vi "Top_Level_Control_Cavities_Pulses_v00.vi"() -> ()   [LabVIEW 2010]
doc: "Provides user interface for `Cavities_Pulse_FPGA_v00.vi'."
uses:
  Strict Type Defs/Control GUI v01.ctl
  Strict Type Defs/Slider and display.ctl
  Strict Type Defs/I16 white control.ctl
  Strict Type Defs/PII Gains.ctl
  Strict Type Defs/I2 gain slider.ctl
  Strict Type Defs/Thresh slider.ctl
  Strict Type Defs/Lock or Hold.ctl
  Strict Type Defs/Scan Freq Slider.ctl
  Strict Type Defs/DC polarity.ctl
  Strict Type Defs/Gains negative vertical.ctl
  <vilib>/userDefined/High Color/nirio_resource_hc.ctl
  Strict Type Defs/Lock Select.ctl
  Strict Type Defs/Scope and Safety.ctl
  Strict Type Defs/Hold All.ctl
  Strict Type Defs/Cavity Extras.ctl
  Strict Type Defs/Pre-Offset.ctl
  Strict Type Defs/Pulse Control.ctl
  <vilib>/rvi/interface/nirviOpenFPGA/nirviOpenFPGA.xnode
  FPGA Bitfiles/PIIphaselocks_FPGATarget_CavitiesPulseFPG_483F4CC6.lvbitx
  <vilib>/rvi/ClientSDK/nirviWhatTheDeviceIsDoing.ctl
  <vilib>/rvi/interface/nirviReadWriteControl/nirviReadWriteControl.xnode
  <vilib>/rvi/interface/common/niFpgaNodeNameForErrorReporting.ctl
  <vilib>/rvi/errors/niLvFpgaWhatHappensToTopLevelVI.ctl
  <vilib>/rvi/interface/nirviMethod/nirviMethod.xnode
  <vilib>/rvi/interface/nirviCloseFPGA/nirviCloseFPGA.xnode
  <vilib>/FPGAPlugInAG/PXI-7833R/niLvFpga_Open_PXI-7833R.vi
  <vilib>/rvi/interface/common/dynamic/niFpgaDynamicAddResources.vi
  <vilib>/Utility/error.llb/Error Cluster From Error Code.vi
  <vilib>/rvi/errors/niLvFpgaAdjustHostInterfaceError.vi
  <vilib>/FPGAPlugInAG/Dynamic/niLvFpga_Close_Dynamic.vi
  NiFpgaLv.dll
panel:
  out "Any Unlocked?":bool=TRUE
  out "Locked?":T1={"OPO A"=FALSE, "OPO B"=FALSE, "MCC"=FALSE, "Doubler"=TRUE}
  in  "Measurement OFF":bool
  in  "watertank":bool
  out "Water Tank":dbl(slide)=-0.29411764705882354 scale=-0.3..0.3
  in  "Stop Pulses":bool
  in  "Pulses":bool
  out "Top Loop Count":i32=272090
  out "Measurment Pulse":bool
  out "HD Pulse":bool
  out "Probe OFF Pulse":bool=TRUE
  out "BS Hold Pulse":bool=TRUE
  in  "stop":bool
  in  "Hold All":T2
  in  "Extra Controls":T3(tab)=enum."Other"
  in  "Scope+Safety":T4={"Safety First"={"lim reset"=FALSE, "no limit"=FALSE, "pos slew rate * dt"=12, "neg slew rate * dt"=-12, "Count(Ticks)"=0}, "Scope IPs"={"Trigger Direction"=enum."minus-plus", "Trigger Delay (ms)"=0.0, "Aquisition Rate (kHz)"=4000.0, "Trigger Offset (V)"=0.0, "Scale Offset"={"Scaling"={"Error signal"=1, "Output"=0, "DC Monitor"=1, "Threshold"=1}, "Offset"={"Error Signal"=0, "Output"=0, "DC Monitor"=0, "Threshold"=0}}}}
  in  "Cavity Extras":T5={"Pre-Offset"={"OPO A"=0.0, "OPO B"=0.0, "MCC"=0.0, "Doubler"=0.0}, "Pre-Offset DC"={"OPO A"=0.0, "OPO B"=0.0, "MCC"=0.0, "Doubler"=0.0}, "I Max value"=2147483647, "I2 Max value"=0, "Scan Offset"={"OPO A"=0.0, "OPO B"=0.0, "MCC"=0.0, "Doubler"=0.0}, "Scan Ampl."={"OPO A"=1000.0, "OPO B"=1000.0, "MCC"=1000.0, "Doubler"=1000.0}, "Scan-PII thresh"={"OPO A"=100, "OPO B"=100, "MCC"=100, "Doubler"=100}, "Re-Scan thresh"={"OPO A"=1, "OPO B"=1, "MCC"=4, "Doubler"=0}}
  out "xy HD A":cluster{i16[], i16[]}(graph)
  in  "XY HD ON":bool
  out "xy HD B":cluster{i16[], i16[]}(graph)
  in  "Pulse Control":T7={"BS Hold Invert"=FALSE, "Probe Invert"=FALSE, "HD Invert"=TRUE, "Measurement Invert"=FALSE, "BS Hold Delay"=0, "Probe Delay"=10, "HD Delay"=25, "Measurement delay"=80, "High Pulse"=4000, "Low Pulse"=-3200, "Sample & Hold Period (uSec)"=500, "BS Hold ON until"=325, "Probe OFF until"=315, "HD ON until"=305, "Measurement ON until"=280, "Loop period (us)"=0}
  out "Cavities Pulse Loop count":i32=247262374
  out "Tick Count Cavities (uSec)":u32=4069594290 caption="Cavities Tick Count (uSec)"
  out "Cavities Control Loop count":i32=2147483647
  in  "offset time":u32=100
  in  "Measurement OFF (uSec)":u32=1100000
  in  "Lock Monitor":T8={"OPO A"=80, "OPO B"=80, "MCC"=80, "Doubler"=0}
  out "PXI Trig 2":bool=TRUE
  out "Cavities error out":errorcluster
  in  "Loop Delays (uSec)":u32=5
  in  "Number of Elements":u32=4095
  in  "Cavities_Pulse_FPGA_v00":T9="RIO0" caption="RIO Device"
  in  "Scope":T10=TRUE
  out "Scope Graph":cluster{dbl[], dbl[]}[](graph)
  in  "Lock Select":T11
  in  "OPO A":T12={"Offset Error"=-0.004322033898305084, "Gain Error"=1, "Offset DC"=0.18926553672316412, "Gain DC"=1, "P Gain"=12, "P Bit Shift"=-7, "I Bit Shift"=-7, "I2 Bit Shift"=-27, "I Gain"=19, "I2 Gain"=0, "Lock Threshold"=66, "Lock"=FALSE, "Hold"=FALSE, "Scan Frequency"=19, "Scan Bit Shift"=-4, "DC negative"=FALSE, "Gains -ve "=FALSE} {"Scan Frequency" scale=1.0..30.0; "I2 Gain" scale=0.0..10.0; "I Gain" scale=0.0..50.0; "P Gain" scale=0.0..50.0; "Offset DC" scale=-5.0..0.5 scale format="%#_5f"; "Offset Error" scale=-0.01..0.005 scale format="%#_5f"}
  in  "OPO B":T12={"Offset Error"=-0.011977401129943503, "Gain Error"=4, "Offset DC"=1.29177966101695, "Gain DC"=1, "P Gain"=14, "P Bit Shift"=-8, "I Bit Shift"=-8, "I2 Bit Shift"=-27, "I Gain"=13, "I2 Gain"=0, "Lock Threshold"=67, "Lock"=FALSE, "Hold"=FALSE, "Scan Frequency"=10, "Scan Bit Shift"=-5, "DC negative"=TRUE, "Gains -ve "=FALSE} {"Scan Frequency" scale=1.0..30.0; "I2 Gain" scale=0.0..10.0; "I Gain" scale=0.0..50.0; "P Gain" scale=0.0..50.0; "Offset DC" scale=-5.1..3.0 scale format="%#_5f"; "Offset Error" scale format="%#_5f"}
  in  "MCC":T12={"Offset Error"=-0.006610169491525424, "Gain Error"=1, "Offset DC"=0.028813559322033905, "Gain DC"=1, "P Gain"=14, "P Bit Shift"=-8, "I Bit Shift"=-11, "I2 Bit Shift"=-27, "I Gain"=11, "I2 Gain"=0, "Lock Threshold"=20, "Lock"=FALSE, "Hold"=FALSE, "Scan Frequency"=10, "Scan Bit Shift"=-4, "DC negative"=TRUE, "Gains -ve "=TRUE} {"Scan Frequency" scale=1.0..30.0; "I2 Gain" scale=0.0..10.0; "I Gain" scale=0.0..50.0; "P Gain" scale=0.0..50.0; "Offset DC" scale=-0.1..0.2 scale format="%#_5f"; "Offset Error" scale=-0.02..0.01 scale format="%#_5f"}
  in  "Doubler":T12={"Offset Error"=-0.011581920903954804, "Gain Error"=1, "Offset DC"=-0.023163841807909608, "Gain DC"=1, "P Gain"=10, "P Bit Shift"=-7, "I Bit Shift"=-8, "I2 Bit Shift"=-27, "I Gain"=21, "I2 Gain"=0, "Lock Threshold"=12, "Lock"=FALSE, "Hold"=FALSE, "Scan Frequency"=8, "Scan Bit Shift"=-5, "DC negative"=FALSE, "Gains -ve "=FALSE} {"Scan Frequency" scale=1.0..30.0; "I2 Gain" scale=0.0..10.0; "I Gain" scale=0.0..50.0; "P Gain" scale=0.0..50.0; "Offset DC" scale=-0.1..0.1 scale format="%#_5f"; "Offset Error" scale=-0.05..0.05 scale format="%#_5f"}
  # "All time values are in micro-seconds"
  # "PII Gains"
  # "Lock"
  # "Error Signal"
  # "Monitor"
  # "Scan"
  # "DC positive"
  # "PII Gains"
  # "Lock"
  # "Error Signal"
  # "Monitor"
  # "Scan"
  # "DC positive"
  # "PII Gains"
  # "Lock"
  # "Error Signal"
  # "Monitor"
  # "Scan"
  # "DC positive"
  # "PII Gains"
  # "Lock"
  # "Error Signal"
  # "Monitor"
  # "Scan"
  # "DC positive"
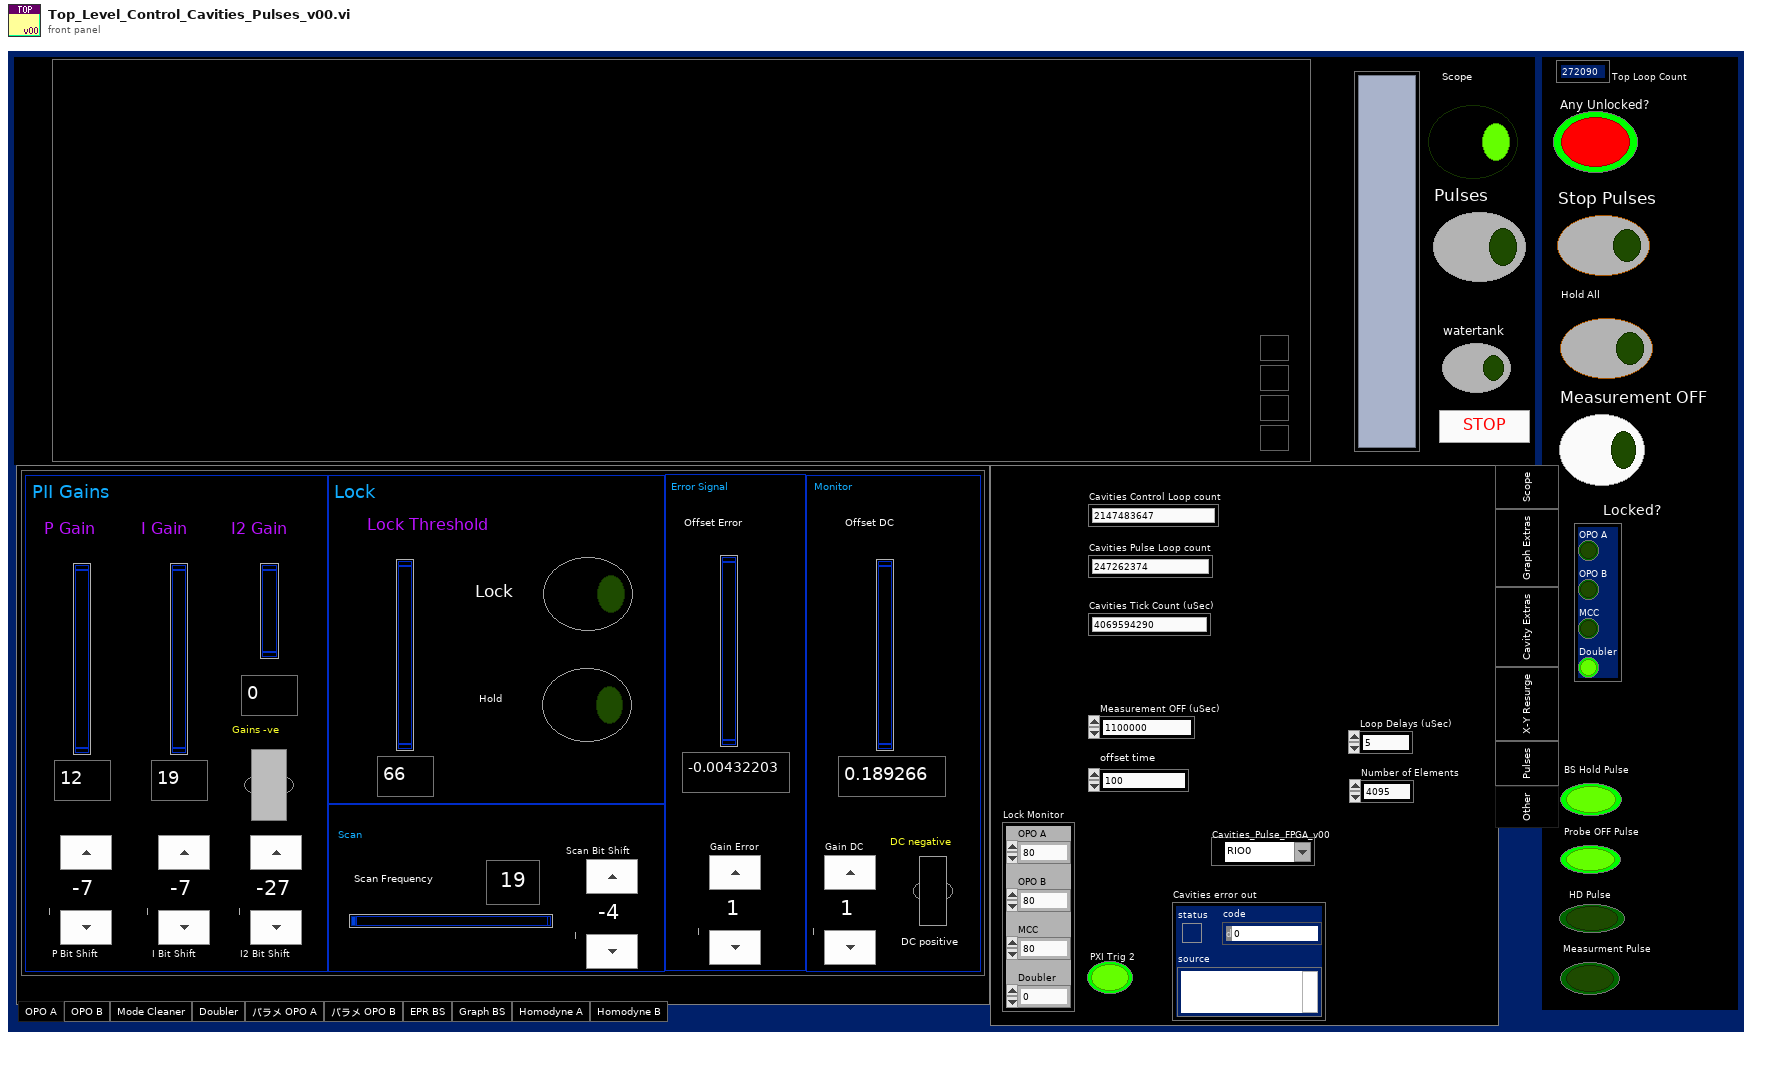
[diagram p1: front panel]
types:
  T1 = cluster{"OPO A":bool, "OPO B":bool, "MCC":bool, "Doubler":bool}
  T2 = typedef "Hold All.ctl" = bool
  T3 = enum32{"Scope", "Graph Extras", "Cavity Extras", "X-Y Resurge", "Pulses", "Other"}
  T4 = typedef "Scope and Safety.ctl" = cluster{"Safety First":cluster{"lim reset":bool, "no limit":bool, "pos slew rate * dt":i16, "neg slew rate * dt":i16, "Count(Ticks)":u32}, "Scope IPs":cluster{"Trigger Direction":enum8{"either", "minus-plus", "plus-minus"}, "Trigger Delay (ms)":dbl, "Aquisition Rate (kHz)":dbl, "Trigger Offset (V)":dbl, "Scale Offset":cluster{"Scaling":cluster{"Error signal":i16, "Output":i16, "DC Monitor":i16, "Threshold":i16}, "Offset":cluster{"Error Signal":i16, "Output":i16, "DC Monitor":i16, "Threshold":i16}}}}
  T5 = typedef "Cavity Extras.ctl" = cluster{"Pre-Offset":T6, "Pre-Offset DC":T6, "I Max value":i32, "I2 Max value":i32, "Scan Offset":T6, "Scan Ampl.":T6, "Scan-PII thresh":cluster{"OPO A":i16, "OPO B":i16, "MCC":i16, "Doubler":i16}, "Re-Scan thresh":cluster{"OPO A":i16, "OPO B":i16, "MCC":i16, "Doubler":i16}}
  T6 = typedef "Pre-Offset.ctl" = cluster{"OPO A":dbl, "OPO B":dbl, "MCC":dbl, "Doubler":dbl}
  T7 = typedef "Pulse Control.ctl" = cluster{"BS Hold Invert":bool, "Probe Invert":bool, "HD Invert":bool, "Measurement Invert":bool, "BS Hold Delay":u32, "Probe Delay":u32, "HD Delay":u32, "Measurement delay":u32, "High Pulse":i16, "Low Pulse":i16, "Sample & Hold Period (uSec)":u32, "BS Hold ON until":u32, "Probe OFF until":u32, "HD ON until":u32, "Measurement ON until":u32, "Loop period (us)":u16}
  T8 = cluster{"OPO A":i16, "OPO B":i16, "MCC":i16, "Doubler":i16}
  T9 = typedef "nirio_resource_hc.ctl" = tag
  T10 = typedef "Lock or Hold.ctl" = bool
  T11 = typedef "Lock Select.ctl" = enum32{"OPO A", "OPO B", "Mode Cleaner", "Doubler", "パラメ OPO A", "パラメ OPO B", "EPR BS", "Graph BS", "Homodyne A", "Homodyne B"}
  T12 = typedef "Control GUI v01.ctl" = cluster{"Offset Error":T13, "Gain Error":T14, "Offset DC":T13, "Gain DC":T14, "P Gain":T15, "P Bit Shift":T14, "I Bit Shift":T14, "I2 Bit Shift":T14, "I Gain":T15, "I2 Gain":T16, "Lock Threshold":T17, "Lock":T10, "Hold":T10, "Scan Frequency":T18, "Scan Bit Shift":T14, "DC negative":T19, "Gains -ve ":T20}
  T13 = typedef "Slider and display.ctl" = dbl
  T14 = typedef "I16 white control.ctl" = i16
  T15 = typedef "PII Gains.ctl" = i32
  T16 = typedef "I2 gain slider.ctl" = i32
  T17 = typedef "Thresh slider.ctl" = i16
  T18 = typedef "Scan Freq Slider.ctl" = u16
  T19 = typedef "DC polarity.ctl" = bool
  T20 = typedef "Gains negative vertical.ctl" = bool
  T21 = typedef "niFpgaNodeNameForErrorReporting.ctl" = enum16{"Open FPGA VI Reference", "Read/Write Control", "Invoke Method: Abort", "Invoke Method: Acknowledge IRQ", "Invoke Method: Download", "Invoke Method: FIFO.Configure", "Invoke Method: FIFO.Read", "Invoke Method: FIFO.Start", "Invoke Method: FIFO.Stop", "Invoke Method: FIFO.Write", "Invoke Method: Reset", "Invoke Method: Run", "Invoke Method: Wait on IRQ", "Close FPGA VI Reference"}
  T22 = typedef "niLvFpgaWhatHappensToTopLevelVI.ctl" = enum16{"top level VI scripted behind XNode", "top level VI inlined behind XNode"}
  T23 = typedef "Top Level Control.ctl" = cluster{"Safety First":T24, "Error scale":T25, "Lock Select":enum32{"OPO A", "OPO B", "Mode Cleaner", "Doubler", "パラメ OPO A", "パラメ OPO B", "EPR Beamsplitter", "Graph Beamsplitter", "Homodyne A", "Homodyne B"}, "Controls":cluster{"OPO A":T26, "OPO B":T26, "MCC":T26, "Doubler":T26}, "Scope IPs":cluster{"Trigger Direction":enum8{"either", "minus-plus", "plus-minus"}, "Trigger Delay (ms)":dbl, "Aquisition Rate (kHz)":dbl, "Trigger Offset (V)":dbl, "Trigger Channel":i32, "Channel Selector":cluster{"Channel 1":i32, "Channel 2":i32, "Channel 3":i32, "Channel 4":i32}, "Scale Offset":cluster{"Scaling":cluster{"Scan Scale":i16, "Scan Scale 2":i16, "Scan Scale 3":i16, "Scan Scale 4":i16}, "Offset":cluster{"Scan Offset":i16, "Scan Offset 2":i16, "Scan Offset 3":i16, "Scan Offset 4":i16}}}, "PII A":T31, "PII B":T31, "PII MCC":T31, "PII Doubler":T31, "Peak Depth (%)":cluster{"Peak Depth (%) 1":i16, "Peak Depth (%) 2":i16, "Peak Depth (%) 3":i16, "Peak Depth (%) 4":i16}}
  T24 = typedef "Safety First.ctl" = cluster{"lim reset":bool, "no limit":bool, "pos slew rate * dt":i16, "neg slew rate * dt":i16, "Hold All":bool, "Count(Ticks)":u32}
  T25 = typedef "Error_Scale.ctl" = cluster{"Bit Shift":cluster{"Bit Shift 1":i16, "Bit Shift 2":i16, "Bit Shift 3":i16, "Bit Shift 4":i16, "Bit Shift 5":i16, "Bit Shift 6":i16, "Bit Shift 7":i16, "Bit Shift 8":i16}, "Pre-Offset":cluster{"Pre-Offset 1":i16, "Pre-Offset 2":i16, "Pre-Offset 3":i16, "Pre-Offset 4":i16, "Pre-Offset 5":i16, "Pre-Offset 6":i16, "Pre-Offset 7":i16, "Pre-Offset 8":i16}, "Post-Offset ":cluster{"Offset 1":i16, "Offset 2":i16, "Offset 3":i16, "Offset 4":i16, "Offset 5":i16, "Offset 6":i16, "Offset 7":i16, "Offset 8":i16}, "Gains":cluster{"Gain 1":i16, "Gain 2":i16, "Gain 3":i16, "Gain 4":i16, "Gain 5":i16, "Gain 6":i16, "Gain 7":i16, "Gain 8":i16}, "Polarity DC":cluster{"False 1":bool, "False 2":bool, "False 3":bool, "False 4":bool, "DC x -1":bool, "DC x -1 2":bool, "DC x -1 3":bool, "DC x -1 4":bool}}
  T26 = typedef "Control GUI v00.ctl" = cluster{"Pre Offset":T13, "Offset":T13, "Gain":T14, "Bit Shift":T14, "Pre Offset 2":T13, "Offset 2":T13, "Gain 2":T14, "Bit Shift 2":T14, "P Gain":T15, "P Bit Shift":T14, "I Bit Shift":T14, "I2 Bit Shift":T14, "I Gain":T15, "I2 Gain":T15, "Lock Threshold":T17, "Lock":T10, "Hold":T10, "Scan Offset (mV)":T27, "Scan Amplitude (mV)":T27, "Scan Frequency":T28, "Scan Bit Shift":T14, "DC x -1":T19, "Gains x -1":T29, "I Max value":T30, "I2 Max value":T30}
  T27 = typedef "Scan Amp slider.ctl" = dbl
  T28 = typedef "Scan Frequency.ctl" = u16
  T29 = typedef "Gains negative.ctl" = bool
  T30 = typedef "I max value.ctl" = i16
  T31 = typedef "Top Level PII.ctl" = cluster{"Lock":bool, "Hold":bool, "P Gain":i16, "P BS":i16, "I Gain":i16, "I BS":i16, "I2 G":i16, "I2 BS":i16, "Scan Amp":i16, "Scan Off":i16, "Scan FS":u16, "SFS BS":i16, "I Max value":i16, "I2 Max value":i16}
  T32 = cluster{"Trigger Direction":enum8{"either", "minus-plus", "plus-minus"}, "Trigger Delay (ms)":dbl, "Aquisition Rate (kHz)":dbl, "Trigger Offset (V)":dbl, "Scale Offset":cluster{"Scaling":cluster{"Scan Scale":i16, "Scan Scale 2":i16, "Scan Scale 3":i16, "Scan Scale 4":i16}, "Offset":cluster{"Scan Offset":i16, "Scan Offset 2":i16, "Scan Offset 3":i16, "Scan Offset 4":i16}}}
  T33 = cluster{"PII In 1":cluster{"Lock":bool, "Hold":bool, "P Gain":i32, "P BS":i16, "I Gain":i32, "I BS":i16, "I2 G":i32, "I2 BS":i16, "Scan Amp":i16, "Scan Off":i16, "Scan FS":u16, "SFS BS":i16, "I Max value":i32, "I2 Max value":i32, "Scope.Offset":i16, "Trigger Direction":enum8{"either", "minus-plus", "plus-minus"}, "Scan-PII thresh":i16}, "PII In 2":cluster{"Lock":bool, "Hold":bool, "P Gain":i32, "P BS":i16, "I Gain":i32, "I BS":i16, "I2 G":i32, "I2 BS":i16, "Scan Amp":i16, "Scan Off":i16, "Scan FS":u16, "SFS BS":i16, "I Max value":i32, "I2 Max value":i32, "Scope.Offset":i16, "Trigger Direction":enum8{"either", "minus-plus", "plus-minus"}, "Scan-PII thresh":i16}, "PII In 3":cluster{"Lock":bool, "Hold":bool, "P Gain":i32, "P BS":i16, "I Gain":i32, "I BS":i16, "I2 G":i32, "I2 BS":i16, "Scan Amp":i16, "Scan Off":i16, "Scan FS":u16, "SFS BS":i16, "I Max value":i32, "I2 Max value":i32, "Scope.Offset":i16, "Trigger Direction":enum8{"either", "minus-plus", "plus-minus"}, "Scan-PII thresh":i16}, "PII In 4":cluster{"Lock":bool, "Hold":bool, "P Gain":i32, "P BS":i16, "I Gain":i32, "I BS":i16, "I2 G":i32, "I2 BS":i16, "Scan Amp":i16, "Scan Off":i16, "Scan FS":u16, "SFS BS":i16, "I Max value":i32, "I2 Max value":i32, "Scope.Offset":i16, "Trigger Direction":enum8{"either", "minus-plus", "plus-minus"}, "Scan-PII thresh":i16}, "Safety First":cluster{"lim reset":bool, "no limit":bool, "pos slew rate * dt":i16, "neg slew rate * dt":i16, "Hold All":bool, "Count(Ticks)":u32}, "Error scale":cluster{"Pre-Offset":cluster{"Pre-Offset 1":i16, "Pre-Offset 2":i16, "Pre-Offset 3":i16, "Pre-Offset 4":i16, "Pre-Offset 5":i16, "Pre-Offset 6":i16, "Pre-Offset 7":i16, "Pre-Offset 8":i16}, "Post-Offset ":cluster{"Offset 1":i16, "Offset 2":i16, "Offset 3":i16, "Offset 4":i16, "Offset 5":i16, "Offset 6":i16, "Offset 7":i16, "Offset 8":i16}, "Gains":cluster{"Gain 1":i16, "Gain 2":i16, "Gain 3":i16, "Gain 4":i16, "Gain 5":i16, "Gain 6":i16, "Gain 7":i16, "Gain 8":i16}, "Polarity DC":cluster{"False 1":bool, "False 2":bool, "False 3":bool, "False 4":bool, "DC x -1":bool, "DC x -1 2":bool, "DC x -1 3":bool, "DC x -1 4":bool}}, "Lock Thresh":cluster{"OPO A":i16, "OPO B":i16, "MCC":i16, "Doubler":i16}, "Re-Scan Thresh":cluster{"OPO A":i16, "OPO B":i16, "MCC":i16, "Doubler":i16}}
  T34 = cluster{"Trigger Direction":enum8{"either", "minus-plus", "plus-minus"}, "Delay":u32, "Aquisition Rate (Ticks)":u32, "Offset":i16, "Channel":i32, "Channel Selector":cluster{"Channel 1":i32, "Channel 2":i32, "Channel 3":i32, "Channel 4":i32}}
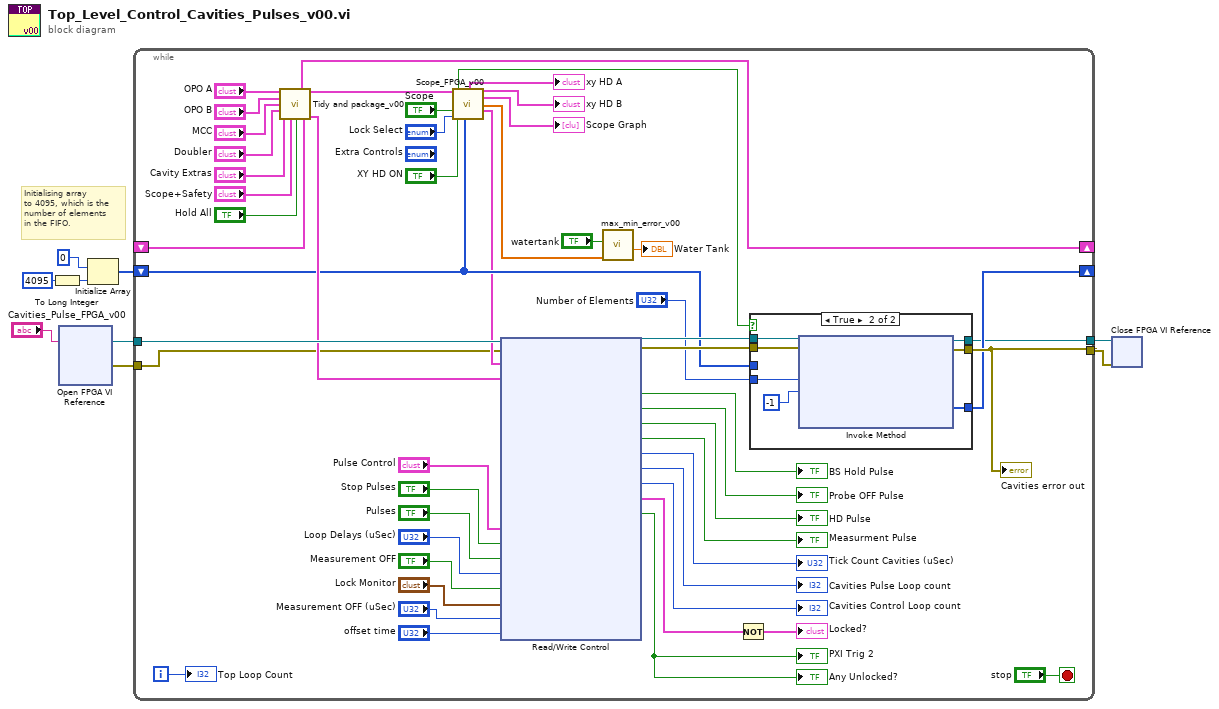
[diagram p0: block diagram]
diagram:
  # "Initialising array\nto 4095, which is the\nnumber of elements\nin the FIFO."
  n1 = To Long Integer(number=4095) -> (32bit integer=w6:i32)
  n2 = xnode "Open FPGA VI Reference"("resource name"="Cavities_Pulse_FPGA_v00") -> ("FPGA VI Reference Out"=w8:refnum<k20>, "error out"=w7:errorcluster)  [unwired: 1 in]
  n3 = Initialize Array(u64 0 ("element"), w6) -> (w3:u64[])
  n4 = while {
    tunnel: w8 -> [w60]
    tunnel: w7 -> [w30]
    tunnel: [w56] -> w1
    shift-right: [w54] -> _
    shift-left: w3 -> [w38]
    shift-right: [w10] -> _
    shift-left: _ -> [w11]
    tunnel: [w53] -> w2
    i -> [w58]
    stop <- "stop" stop-if-true
    n5 = call "Tidy and package_v00.vi"("OPO A"="OPO A", "OPO B"="OPO B", "MCC"="MCC", "Doubler"="Doubler", "PII Controls (-1)"=w11, "Cavity Extras"="Cavity Extras", "Scope+Safety"="Scope+Safety", "Hold All"="Hold All") -> ("PII Controls cluster"=w10:T23, "Scope IPs"=w45:T32, "Control to FPGA"=w48:T33)  [unwired: 5 in]
    n6 = call "Scope_FPGA_v00.vi"("Scope IPs"=w45, "Scope"="Scope", "Lock Select"="Lock Select", "Cavities Data"=w38, "XY HD ON"="XY HD ON") -> ("xy HD A"=→"xy HD A":cluster{i16[], i16[]}, "xy HD B"=→"xy HD B":cluster{i16[], i16[]}, "Scope OP Graph"=→"Scope Graph":cluster{dbl[], dbl[]}[], "Scope Cavities ON"=w12:bool, "error"=w24:dbl[], "Scope Cavities"=w33:T34)  [unwired: 3 in, 2 out]
    n7 = xnode "Read/Write Control"("FPGA VI Reference In"=w60, "error in"=w30, "Scope"=w33, "Control"=w48, "Pulse Control"="Pulse Control", "stop pulse loop"="Stop Pulses", "Pulse Loop On"="Pulses", "Cavities Delay(uSec)"="Loop Delays (uSec)", "Measurement OFF"="Measurement OFF", "Lock Monitor"="Lock Monitor", "Measurement OFF (uSec)"="Measurement OFF (uSec)", "offset time"="offset time") -> ("FPGA VI Reference Out"=w55:refnum<k20>, "error out"=w57:errorcluster, "BS Hold Pulse"=→"BS Hold Pulse":bool, "Probe OFF Pulse"=→"Probe OFF Pulse":bool, "HD Pulse"=→"HD Pulse":bool, "Measurment Pulse"=→"Measurment Pulse":bool, "Tick Count(uSec)"=→"Tick Count Cavities (uSec)":u32, "Pulse Loop count"=→"Cavities Pulse Loop count":i32, "Control Loop count"=→"Cavities Control Loop count":i32, "Unlocked?(T=yes)"=w15:T1, "PXI Trig 2"=→"PXI Trig 2" →"Any Unlocked?":bool)
    n8 = call "max_min_error_v00.vi"("Array"=w24, "maxmin"="watertank") -> ("x+y"=→"Water Tank":dbl)  [unwired: 7 in, 2 out]
    n9 = Not(x=w15) -> (.not. x?=→"Locked?":T1)
    n10 = case shown="True" w12 {
      tunnel: w57 -> [w63 w70]
      tunnel: [w63 w69] -> w56
      tunnel: w55 -> [w62 w68]
      tunnel: [w62 w67] -> w53
      tunnel: [w61 w66] -> w54
      tunnel: w38 -> [w61 _]
      tunnel: "Number of Elements" -> [_ w64]
      frame False {
      }
      frame True {
        n11 = xnode "Invoke Method"("FPGA VI Reference In"=w68, "error in"=w70, "Number of Elements"=w64, "Timeout (ms)"=-1) -> ("FPGA VI Reference Out"=w67:refnum<k20>, "error out"=w69:errorcluster, "Data"=w66:u64[])  [unwired: 1 out]
      }
    }
    "Cavities error out" <- w56
    "Top Loop Count" <- w58
  }
  n12 = xnode "Close FPGA VI Reference"("FPGA VI Reference In"=w2, "error in"=w1) -> ()  [unwired: 1 out]
